vi "setting.vi"(10 "value":dbl, 11 "setting":string) -> (3 "write":string)   [LabVIEW 2019]
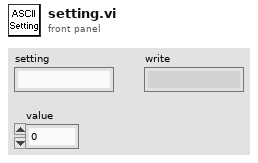
[diagram p1: front panel]
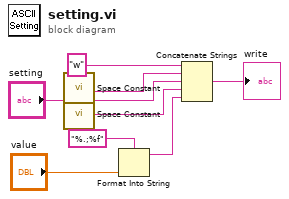
[diagram p0: block diagram]
diagram:
  n1 = call <vilib>:"Space Constant.vi"() -> ("String"=w3:string)
  n2 = call <vilib>:"Space Constant.vi"() -> ("String"=w1:string)
  n3 = Format Into String(format string="%.;%f", "value") -> (resulting string=w6:string)  [unwired: 2 in, 1 out]
  n4 = Concatenate Strings("w" ("write buffer"), w3, "setting", w1, w6) -> (→"write":string)
